vi "Graph_signal.vi"(8 "error in (no error)":errorcluster, 10 "Grafica":waveform(dbl)(graph), 11 "GUI_Actor in":refnum<class "GUI_Actor.lvclass">) -> (0 "error out":errorcluster, 3 "GUI_Actor out":refnum<class "GUI_Actor.lvclass">)   [LabVIEW 2019, in "GUI_Actor.lvlib" / "GUI_Actor.lvclass"]
uses:
  GUI_Actor.lvclass
  GUI_Actor.lvclass/GUI_Actor.ctl
  Logging_txt/Logging_txt Messages/Save_data_txt Msg/Save_data_txt Msg.lvclass/Save_data_txt Msg.ctl
  <vilib>/ActorFramework/Message Enqueuer/Message Enqueuer.lvclass/Message Enqueuer.ctl
  <vilib>/ActorFramework/Message Enqueuer/Enqueue.vi
  Logging_txt/Logging_txt Messages/Save_data_txt Msg/Save_data_txt Msg.lvclass
  C:/Program Files/National Instruments/LabVIEW 2019/vi.lib/ActorFramework/Message/Message.lvclass
  <vilib>/ActorFramework/Message Priority Queue/Priority Enqueue.vi
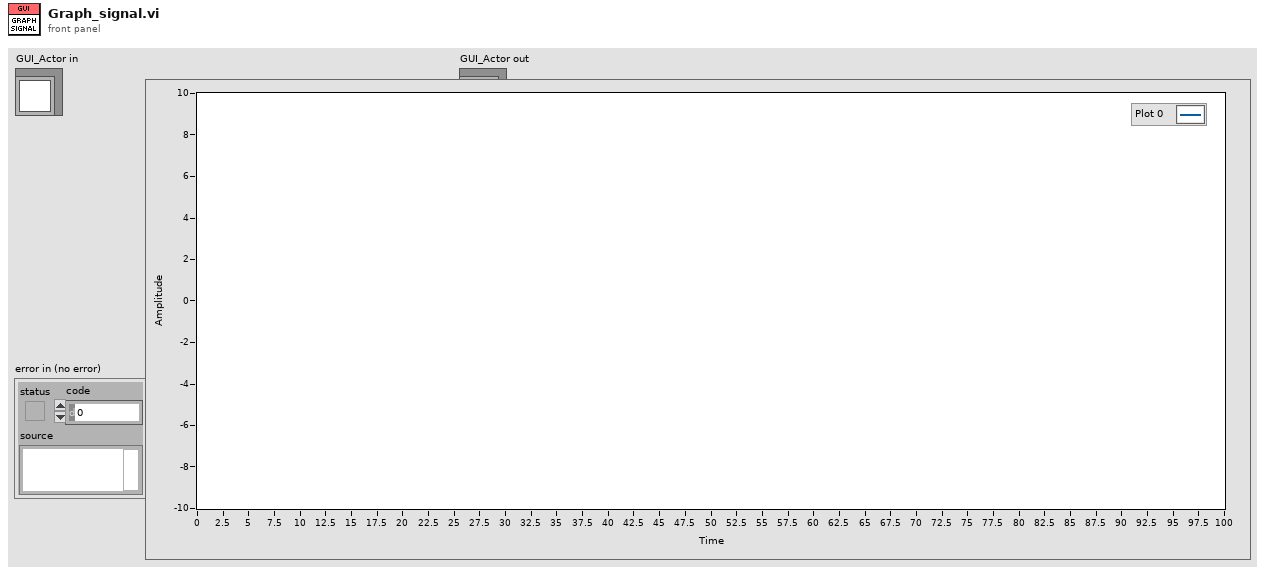
[diagram p1: front panel]
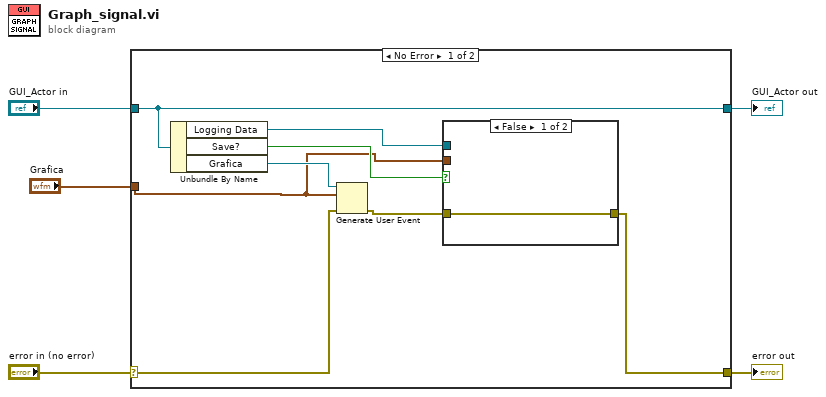
[diagram p0: block diagram]
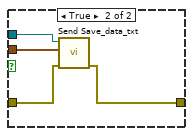
[diagram p2: hidden frame]
diagram:
  n1 = case shown="No Error" "error in (no error)" {
    selector: "error in (no error)" -> [w11 w20]
    tunnel: [w6 w20] -> w4
    tunnel: [w13 w19] -> w2
    tunnel: "GUI_Actor in" -> [w13 w19]
    tunnel: "Grafica" -> [w8 _]
    frame No Error {
      n2 = Unbundle By Name(w13) -> ("Logging Data"=w9:refnum<class "Message Enqueuer.lvclass">, "Save?"=w10:bool, "Grafica"=w12:refnum<user-event>)
      n3 = Generate User Event(user event=w12, event data cluster=w8, error in=w11) -> (error out=w7:errorcluster)  [unwired: 1 in, 1 out]
      n4 = case shown="False" w10 {
        tunnel: w9 -> [_ w18]
        tunnel: w8 -> [_ w17]
        tunnel: w7 -> [w14 w16]
        tunnel: [w14 w15] -> w6
        frame False {
        }
        frame True {
          n5 = call "Send Save_data_txt.vi"("error in (no error)"=w16, "Grafica"=w17, "Message Enqueuer"=w18) -> ("error out"=w15:errorcluster)  [unwired: 7 in, 1 out]
        }
      }
    }
    frame Error {
    }
  }
  "error out" <- w4
  "GUI_Actor out" <- w2
